vi "Calculate Line Reciprocal.vi"(10 "P2":T1, 11 "P1":T1) -> (3 "Column Pixels Per Row":sgl)   [LabVIEW 2022 SP3, in "Raster.lvlib"]
uses:
  Raster.lvlib
  Point 2D.ctl
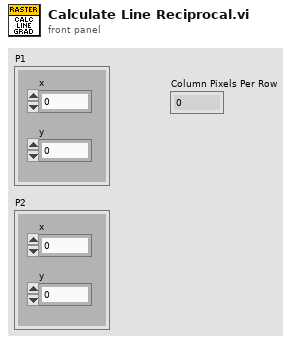
[diagram p1: front panel]
types:
  T1 = typedef "Raster.lvlib/Point 2D.ctl" = cluster{"x":i32, "y":i32}
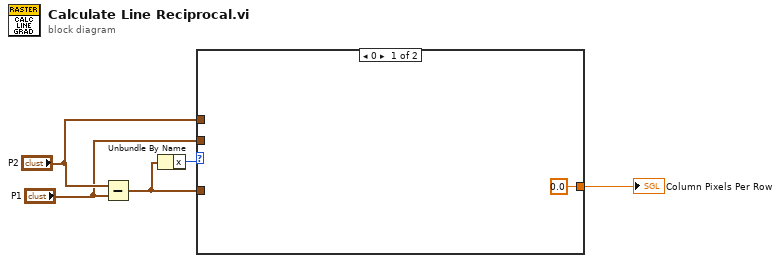
[diagram p0: block diagram]
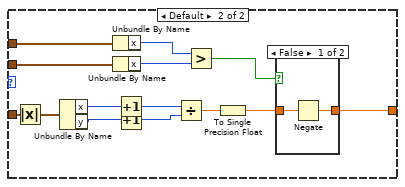
[diagram p2: hidden frame]
diagram:
  n1 = Subtract(x="P2", y="P1") -> (x-y=w2:T1)
  n2 = Unbundle By Name(w2) -> ("x"=w1:i32)
  n3 = case shown="0" w1 {
    tunnel: w2 -> [_ w20]
    tunnel: "P2" -> [_ w13]
    tunnel: "P1" -> [_ w12]
    tunnel: [sgl 0.0 w7] -> w3
    frame 0 {
    }
    frame Default {
      n4 = Absolute Value(x=w20) -> (abs(x)=w14:T1)
      n5 = Unbundle By Name(w14) -> ("x"=w19:i32, "y"=w18:i32)
      n6 = Unbundle By Name(w13) -> ("x"=w11:i32)
      n7 = Unbundle By Name(w12) -> ("x"=w10:i32)
      n8 = Increment(x=w19) -> (x+1=w17:i32)
      n9 = Increment(x=w18) -> (x+1=w16:i32)
      n10 = Divide(x=w17, y=w16) -> (x/y=w15:dbl)
      n11 = Greater?(x=w11, y=w10) -> (0:w9:bool)
      n12 = To Single Precision Float(number=w15) -> (single precision float=w8:sgl)
      n13 = case shown="False" w9 {
        tunnel: w8 -> [w22 w23]
        tunnel: [w21 w23] -> w7
        frame False {
          n14 = Negate(x=w22) -> (-x=w21:sgl)
        }
        frame True {
        }
      }
    }
  }
  "Column Pixels Per Row" <- w3
